vi "Auto Selector.vi"(8 "error in (no error)":errorcluster) -> ()   [LabVIEW 2019]
uses:
  <vilib>/Rock Robotics/Network Tables/NT Read String.vi
  Framework/Robot Global Data.vi
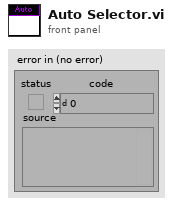
[diagram p1: front panel]
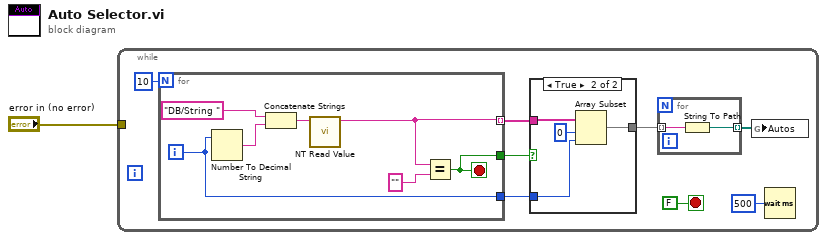
[diagram p0: block diagram]
diagram:
  n1 = while {
    tunnel: "error in (no error)" -> [_]
    stop <- FALSE stop-if-true
    n2 = for {
      N: 10 -> [_]
      tunnel: [w13] -> w7 mode=indexing
      tunnel: [w11] -> w8
      tunnel: [w10] -> w2
      i -> [w10]
      stop <- w11 stop-if-true
      n3 = Number To Decimal String(number=w10) -> (decimal integer string=w15:string)  [unwired: 1 in]
      n4 = Concatenate Strings("DB/String " ("Name"), w15) -> (w14:string)
      n5 = call-poly <vilib>:"NT Read Value.vi"("Name"=w14) -> ("String"=w13:string)  [unwired: 9 in, 1 out]
      n6 = Equal?(x=w13, y="" ("x")) -> (x = y?=w11:bool)
    }
    n7 = case shown="True" w8 {
      tunnel: w7 -> [w17 w19]
      tunnel: [w17 w21] -> w5
      tunnel: w2 -> [_ w18]
      frame False {
      }
      frame True {
        n8 = Array Subset(array=w19, index=0, length=w18) -> (w21:string[])
      }
    }
    n9 = for {
      tunnel: w5 -> [w23] mode=indexing
      tunnel: [w22] -> w4 mode=indexing
      n10 = String To Path(string=w23) -> (path=w22:path)
    }
    n11 = global write "Robot Global Data.vi" "Autos"(w4) -> ()
    n12 = Wait (ms)(milliseconds to wait=u32 500) -> ()  [unwired: 1 out]
  }
